vi "Get Bus Status Section and Channels.vi"(8 "error in":errorcluster, 11 "custom device":T1 format="%.0x") -> (0 "error out":errorcluster, 1 "bus status channels":T1[](array[typedef]) format="%.0x", 2 "bus status section":T1 format="%.0x", 3 "custom device out":T1 format="%.0x", 4 "found":bool)   [LabVIEW 2020, in "AIM MIL-STD-1553 Scripting.lvlib"]
doc: "Gets <b>configuration files section</b> for the specified custom device."
uses:
  AIM MIL-STD-1553 Scripting.lvlib
  <vilib>/NI VeriStand/Custom Device API/Custom Device Item Ref.ctl
  <vilib>/NI VeriStand/Custom Device Tools/Custom Device Utility Library/NI VeriStand - Search for Item by Name.vi
  <vilib>/NI VeriStand/Custom Device Tools/Custom Device Utility Library/Custom Device Utility Library.lvlib
  <vilib>/NI VeriStand/Custom Device Tools/Custom Device Utility Library/NI VeriStand - Search for Item by GUID.vi
  Constants.vi
  <vilib>/NI VeriStand/Custom Device API/Custom Device API.lvlib
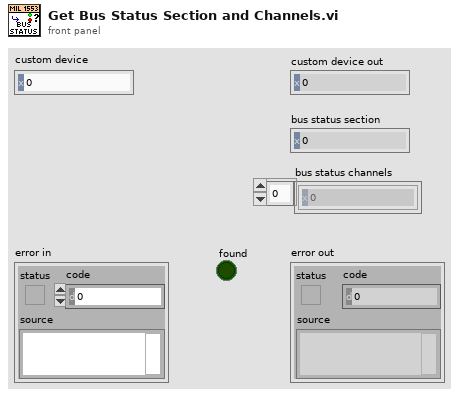
[diagram p1: front panel]
types:
  T1 = typedef "Custom Device API.lvlib/Custom Device Item Ref.ctl" = u64
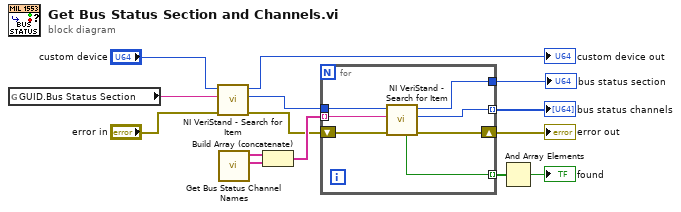
[diagram p0: block diagram]
diagram:
  n1 = global read "Constants.vi" "GUID.Bus Status Section"() -> (w4:string)
  n2 = call-poly <vilib>:"NI VeriStand - Search for Item.vi"("error in"="error in", "Item GUID"=w4, "Section Ref in"="custom device") -> ("error out"=w5:errorcluster, "Item Ref"=w3:T1, "Section Ref out"=→"custom device out":T1)  [unwired: 5 in, 1 out]
  n3 = call "Get Bus Status Channel Names.vi"() -> ("bus status loads"=w12:string[], "bus status counts"=w13:string[])  [unwired: 10 in]
  n4 = Build Array (concatenate)(w13, w12) -> (w11:string[])
  n5 = for {
    tunnel: w3 -> [w21]
    tunnel: [w18] -> w8 mode=indexing
    tunnel: [w17] -> w10 mode=indexing
    tunnel: w11 -> [w16] mode=indexing
    shift-right: [w20] -> w14
    shift-left: w5 -> [w19]
    tunnel: [w15] -> w1
    n6 = call-poly <vilib>:"NI VeriStand - Search for Item.vi"("error in"=w19, "Item Name"=w16, "Section Ref in"=w21) -> ("error out"=w20:errorcluster, "Item Ref"=w18:T1, "Section Ref out"=w15:T1, "Found"=w17:bool)  [unwired: 5 in]
  }
  "error out" <- w14
  "bus status channels" <- w8
  "bus status section" <- w1
  n7 = And Array Elements(Boolean array=w10) -> (logical AND=→"found":bool)
